vi "Set Motion Status.vi"(8 "error in (no error)":errorcluster, 10 "Set Motion Status Data cluster":T1, 11 "Motions in":refnum<class "Motions.lvclass">) -> (0 "error out":errorcluster, 3 "Motions out":refnum<class "Motions.lvclass">)   [LabVIEW 2016, in "Hardware.lvlib" / "Motions.lvlib" / "Motions.lvclass"]
uses:
  <userlib>/Common Components/Hardware/Abstract System/Motions/Motions/Motions.lvclass
  <userlib>/Common Components/Hardware/Abstract System/Motions/Motions/Data_Set Motion Status.ctl
  <userlib>/Common Components/Hardware/Abstract System/Motions/Motions/Motions.lvclass/Motions.ctl
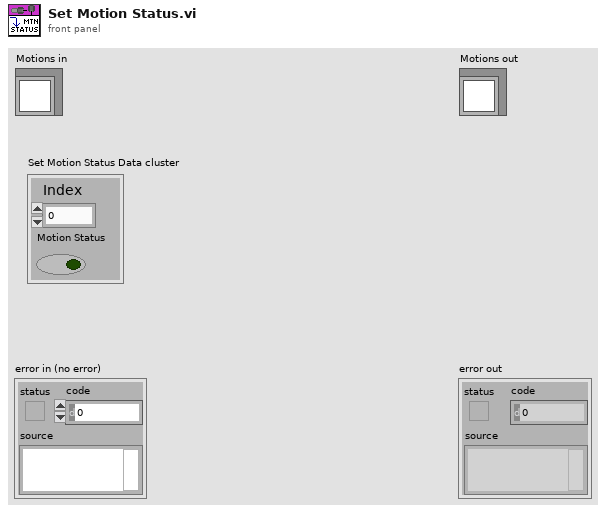
[diagram p1: front panel]
types:
  T1 = typedef "Hardware.lvlib/Motions.lvlib/Motions.lvclass/Data_Set Motion Status.ctl" = cluster{"Index":i32, "Motion Status":bool}
  T2 = typedef "Hardware.lvlib/Motions.lvlib/Motions.lvclass/Motor States.ctl" = cluster{"Connected":bool, "Enabled":bool, "Moving Status":bool, "Soft Moving Status":bool, "Current Pos":dbl, "Target Pos":dbl, "Moving Dir (-1, 0, 1)":i32, "Error Status":bool, "Hard Limit+":bool, "Hard Limit-":bool, "Soft Limit+":bool, "Soft Limit-":bool, "History Dst Stack":refnum<queue>, "Motion Status":bool, "Motion TriggerAction Obj":refnum<class "TriggerAction Q.lvclass">}
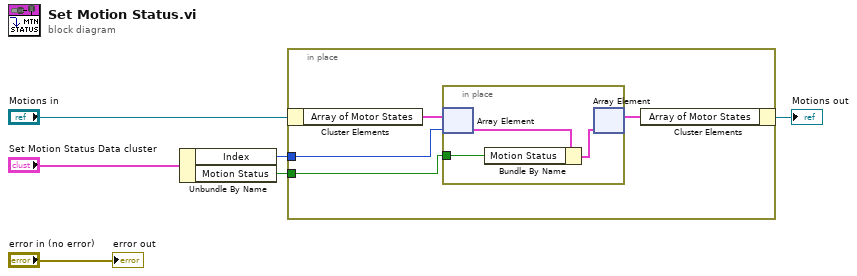
[diagram p0: block diagram]
diagram:
  n1 = Unbundle By Name("Set Motion Status Data cluster") -> ("Index"=w1:i32, "Motion Status"=w2:bool)
  n2 = in-place {
    in-place-border: w2 -> [w8]
    in-place-border: w1 -> [w7]
    n3 = in-place-cluster #1("Motions in") -> ("Array of Motor States"=w10:T2[])
    n4 = in-place {
      in-place-border: w8 -> [w11]
      n5 = in-place-array #2(w10, w7) -> (w13:T2)
      n6 = Bundle By Name(cluster=w13, "Motion Status"=w11) -> (w12:T2)
      n7 = in-place-array #2(w12) -> (w9:T2[])  [unwired: 1 out]
    }
    n8 = in-place-cluster #1("Array of Motor States"=w9) -> (→"Motions out":refnum<class "Motions.lvclass">)
  }
  "error out" <- "error in (no error)"
